vi "Draw.vi"(7 "menu in":refnum<class "menu.lvclass">, 8 "error in (no error)":errorcluster, 11 "icon in":refnum<class "icon.lvclass">) -> (0 "error out":errorcluster, 3 "icon out":refnum<class "icon.lvclass">)   [LabVIEW 2009, in "icon.lvclass"]
uses:
  icon.lvclass
  Menu/menu.lvclass
  icon.lvclass/icon.ctl
  <vilib>/picture/picture.llb/imagedata.ctl
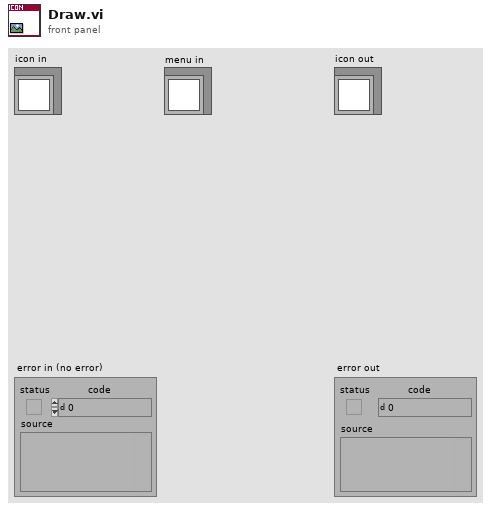
[diagram p1: front panel]
types:
  T1 = typedef "imagedata.ctl" = cluster{"image type":i32, "image depth":i32, "image":u8[], "mask":u8[], "colors":u32[], "Rectangle":cluster{"left":i16, "top":i16, "right":i16, "bottom":i16}}
  T2 = cluster{"left":i16, "top":i16, "right":i16, "bottom":i16}
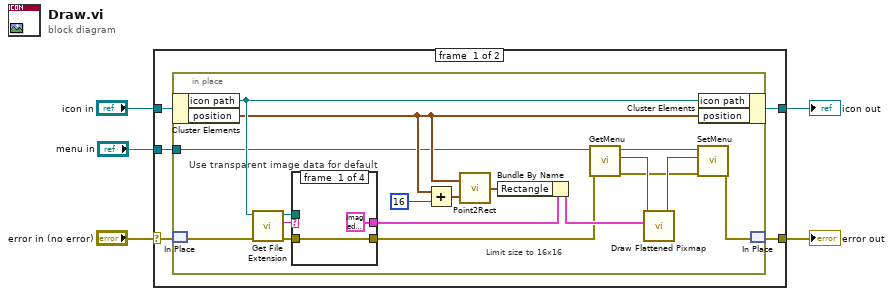
[diagram p0: block diagram]
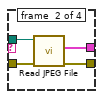
[diagram p2: hidden frame]
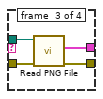
[diagram p3: hidden frame]
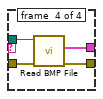
[diagram p4: hidden frame]
diagram:
  n1 = case shown="No Error" "error in (no error)" {
    selector: "error in (no error)" -> [w7 w44]
    tunnel: [w6 w44] -> w2
    tunnel: [w9 w43] -> w4
    tunnel: "icon in" -> [w10 w43]
    tunnel: "menu in" -> [w8 _]
    frame #0 {
      n2 = in-place {
        in-place-border: w8 -> [w19]
        # "Limit size to 16x16"
        n3 = in-place-cluster #1(w10) -> ("icon path"=w28:path, "position"=w21:cluster{"left":u32, "top":u32})
        n4 = in-place-match #2(w7) -> (w27:errorcluster)
        n5 = call <vilib>:"Get File Extension.vi"("error in (no error)"=w27, "file"=w28) -> ("error out"=w24:errorcluster, "lowercase file extension"=w25:string, "dup file"=w26:path)  [unwired: 6 in, 1 out]
        n6 = case "Use transparent image data for default" shown="Default" w25 {
          tunnel: w26 -> [_ w34 w38 w42]
          tunnel: w24 -> [w29 w33 w37 w41]
          tunnel: [w29 w32 w36 w40] -> w14
          tunnel: [T1 {"image type"=0, "image depth"=32, "image"=array[1024 elements], "mask"=[0, 0, 0, 0, 0, 0, 0, 0, 0, 0, 0, 0, 0, 0, 0, 0, 0, 0, 0, 0, 0, 0, 0, 0, 0, 0, 0, 0, 0, 0, 0, 0], "colors"=[], "Rectangle"={"left"=0, "top"=0, "right"=16, "bottom"=16}} ("image data") w31 w35 w39] -> w11
          frame #0 {
          }
          frame #1 {
            n7 = call <vilib>:"Read JPEG File.vi"("error in (no error)"=w33, "path to JPEG file"=w34) -> ("error out"=w32:errorcluster, "image data"=w31:T1)  [unwired: 7 in, 1 out]
          }
          frame #2 {
            n8 = call <vilib>:"Read PNG File.vi"("error in (no error)"=w37, "path to PNG file"=w38) -> ("error out"=w36:errorcluster, "image data"=w35:T1)  [unwired: 7 in, 1 out]
          }
          frame #3 {
            n9 = call <vilib>:"Read BMP File.vi"("error in (no error)"=w41, "path to BMP file"=w42) -> ("error out"=w40:errorcluster, "image data"=w39:T1)  [unwired: 7 in, 1 out]
          }
        }
        n10 = Add(x=w21, y=u32 16 ("left")) -> (x+y=w22:cluster{"left":u32, "top":u32})
        n11 = call <vilib>:"Point2Rect.vi"("point b"=w22, "point a"=w21) -> ("rect"=w20:T2)
        n12 = Bundle By Name(cluster=w11, "Rectangle"=w20) -> (w23:T1)
        n13 = call "GetMenu.vi"("error in (no error)"=w14, "menu in"=w19) -> ("error out"=w15:errorcluster, "menu"=w18:picture, "menu out"=w17:refnum<class "menu.lvclass">)  [unwired: 7 in]
        n14 = call <vilib>:"Draw Flattened Pixmap.vi"("image data"=w23, "picture"=w18) -> ("new picture"=w16:picture)  [unwired: 7 in]
        n15 = call "SetMenu.vi"("error in (no error)"=w15, "menu"=w16, "menu in"=w17) -> ("error out"=w13:errorcluster)  [unwired: 7 in, 1 out]
        n16 = in-place-cluster #1("icon path"=w28, "position"=w21) -> (w9:refnum<class "icon.lvclass">)
        n17 = in-place-match #2(w13) -> (w6:errorcluster)
      }
    }
    frame #1 {
    }
  }
  "icon out" <- w4
  "error out" <- w2
